vi "read_ONE_channel_specify_range.vi"(5 "postDAQ  wait ms":u32=12, 7 "preDAQ  wait ms":u32=25, 8 "error in":T1, 10 "Photodiode Select":u16(ring) items=["PD1", "PD2", "PD3"], 11 "K6517 GPIB Address":string) -> (0 "error out":T1, 2 "data":dbl, 3 "K6517 GPIB Address out":string)   [LabVIEW 2024]
uses:
  <instrlib>/Keithley 6517/Keithley 6517.lvlib
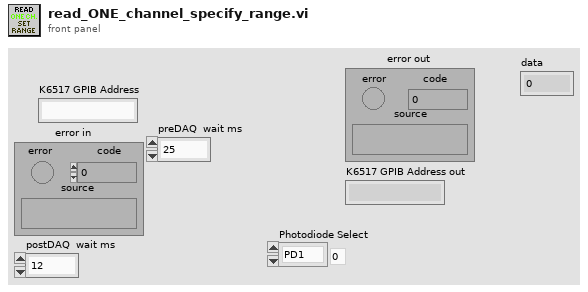
[diagram p1: front panel]
types:
  T1 = cluster{"error":bool, "code":i32, "source":string}
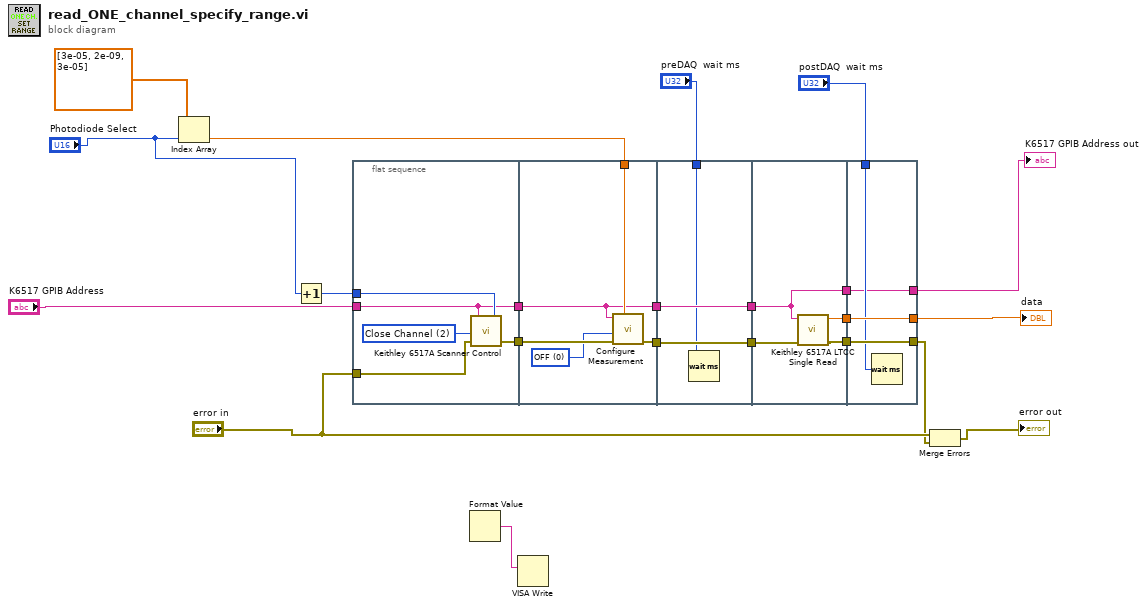
[diagram p0: block diagram]
diagram:
  n1 = Index Array(array=dbl[] [3e-05, 2e-09, 3e-05], index="Photodiode Select") -> (element=w15:dbl)
  n2 = Increment(x="Photodiode Select") -> (x+1=w4:u16)
  n3 = flat-sequence {
    tunnel: w4 -> [w27]
    tunnel: "K6517 GPIB Address" -> [w25]
    tunnel: "error in" -> [w26]
    tunnel: [w25] -> w12
    tunnel: [w24] -> w13
    tunnel: w15 -> [w31]
    tunnel: [w30] -> w11
    tunnel: [w29] -> w10
    tunnel: w13 -> [w33]
    tunnel: w12 -> [w29]
    tunnel: w11 -> [w36]
    tunnel: [w36] -> w9
    tunnel: w10 -> [w35]
    tunnel: [w35] -> w8
    tunnel: "preDAQ  wait ms" -> [w34]
    tunnel: w9 -> [w40]
    tunnel: w8 -> [w37]
    tunnel: [w39] -> w7
    tunnel: [w38] -> w6
    tunnel: [w37] -> w5
    tunnel: [w44] -> w3
    tunnel: w7 -> [w44]
    tunnel: [w43] -> w18
    tunnel: w6 -> [w43]
    tunnel: "postDAQ  wait ms" -> [w42]
    tunnel: [w41] -> w16
    tunnel: w5 -> [w41]
    frame #0 {
      w28 = u16 2 items=["Open All", "Open Channel", "Close Channel", "Scan List"] ("Scanner Control")
      n4 = call "Keithley 6517A Scanner Control.vi"("Open / Close Internal Scanner Channel"=w27, "error in"=w26, "Scanner Control"=w28, "GPIB address"=w25) -> ("error out"=w24:T1)  [unwired: 1 in]
    }
    frame #1 {
      w32 = 0 items=["OFF", "ON", "ONCE"] ("Auto Range (1: ON)")
      n5 = call <instrlib>:"Configure Measurement.vi"("Auto Range Value (2.0000000E+2)"=w31, "error in (no error)"=w33, "Auto Range (1: ON)"=w32, "VISA resource name"=w29) -> ("error out"=w30:errorcluster)  [unwired: 6 in, 1 out]
    }
    frame #2 {
      n6 = Wait (ms)(milliseconds to wait=w34) -> ()  [unwired: 1 out]
    }
    frame #3 {
      n7 = call "Keithley 6517A LTCC Single Read.vi"("error in"=w40, "GPIB address"=w37) -> ("error out"=w39:T1, "measurement"=w38:dbl)  [unwired: 2 in, 6 out]
    }
    frame #4 {
      n8 = Wait (ms)(milliseconds to wait=w42) -> ()  [unwired: 1 out]
    }
  }
  n9 = Format Value() -> (output string=w1:string)  [unwired: 3 in]
  n10 = VISA Write(write buffer=w1) -> (VISA resource name=w2:refnum<visa-resource-name>)  [unwired: 1 in, 3 out]
  n11 = Merge Errors("error in", w3) -> (→"error out":errorcluster)
  "data" <- w18
  "K6517 GPIB Address out" <- w16
